vi "PrepareRollToPassReceiverGoToTactic.vi"(7 "first call":bool, 8 "error in (no error)":errorcluster, 9 "Game in":refnum<class "Game.lvclass">, 10 "Robot":refnum<class "Robot.lvclass">, 11 "PrepareRollToPassReceiverGoToTactic in":refnum<class "PrepareRollToPassReceiverGoToTactic.lvclass">) -> (0 "error out":errorcluster, 2 "Robot out":refnum<class "Robot.lvclass">, 3 "PrepareRollToPassReceiverGoToTactic out":refnum<class "PrepareRollToPassReceiverGoToTactic.lvclass">)   [LabVIEW 2023, in "PrepareRollToPassReceiverGoToTactic.lvclass"]
uses:
  PrepareRollToPassReceiverGoToTactic.lvclass
  Robot_class/Robot.lvclass
  Game_class/Game.lvclass
  Robot_class/tactics.ctl
  Tactic_class/Tactic.lvclass/Tactic.ctl
  Skillbook_class/Skillbook.lvclass/Skillbook.ctl
  Game_class/Game.lvclass/Game.ctl
  Object_class/Object.lvclass/Object.ctl
  Robot_class/Robot.lvclass/Robot.ctl
  PrepareRollToPassReceiverGoToTactic.lvclass/PrepareRollToPassReceiverGoToTactic.ctl
  <vilib>/Analysis/_algsub.llb/Real Vector Norm.vi
  Game_class/Read BallRef.vi
  Game_class/Read FieldRef.vi
  Object_class/Read x.vi
  Object_class/Read y.vi
  Skillbook_class/Read GoToSkill.vi
  Robot_class/Read orientation.vi
  Robot_class/Read dest_x.vi
  Robot_class/Read dest_y.vi
  Robot_class/Read dest_orientation.vi
  Tactic_class/Read Skillbook.vi
  Robot_class/Write tactic.vi
  Write States.vi
  Ball_class/Ball.lvclass
  Skillbook_class/Skillbook.lvclass
  Field_class/Field.lvclass
  GoToSkill_class/GoToSkill.lvclass
  <vilib>/Analysis/NI_AALPro.lvlib
panel:
  out "x .or. y?":bool
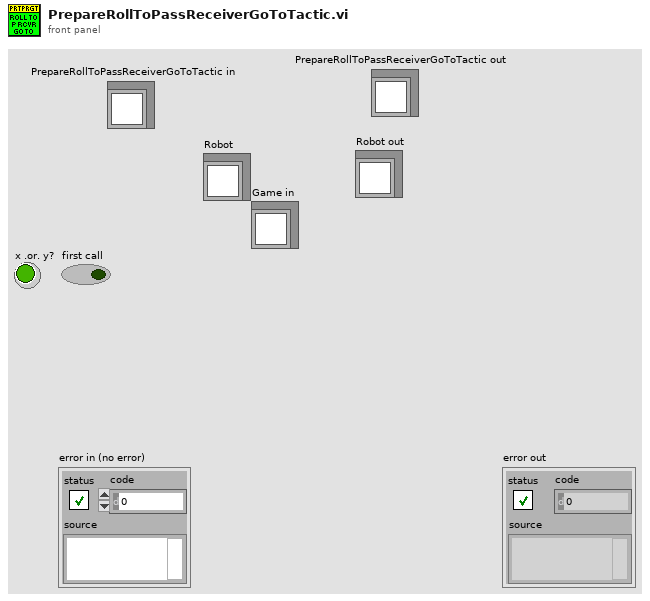
[diagram p1: front panel]
types:
  T1 = typedef "tactics.ctl" = enum16{"ReceivePassInFuturePoint", "Roller", "PrepareRollToPassRollerGoTo", "PrepareRollToPassReceiverGoTo", "WaitRoll", "PositionToRoll", "PenaltyAttacker", "PassObserver", "PenaltyDefense", "TableReceiverTactic", "Test", "DefendGoal", "Marker", "FollowAttacker", "DefendArea", "Shoot", "AttackerAimGoal", "AttackerBallOutOfField", "AttackerBlock", "AttackerStop", "Duelist", "Halt", "ZigZag", "GoTo", "Timeout", "KickToPassReceiver", "PositionToReceivePass", "DefendAreaVSS", "DefendGoalVSS", "KickVSS", "AttackVSS", "DispBallVSS", "PenaltyAttackVSS", "WaitPass"}
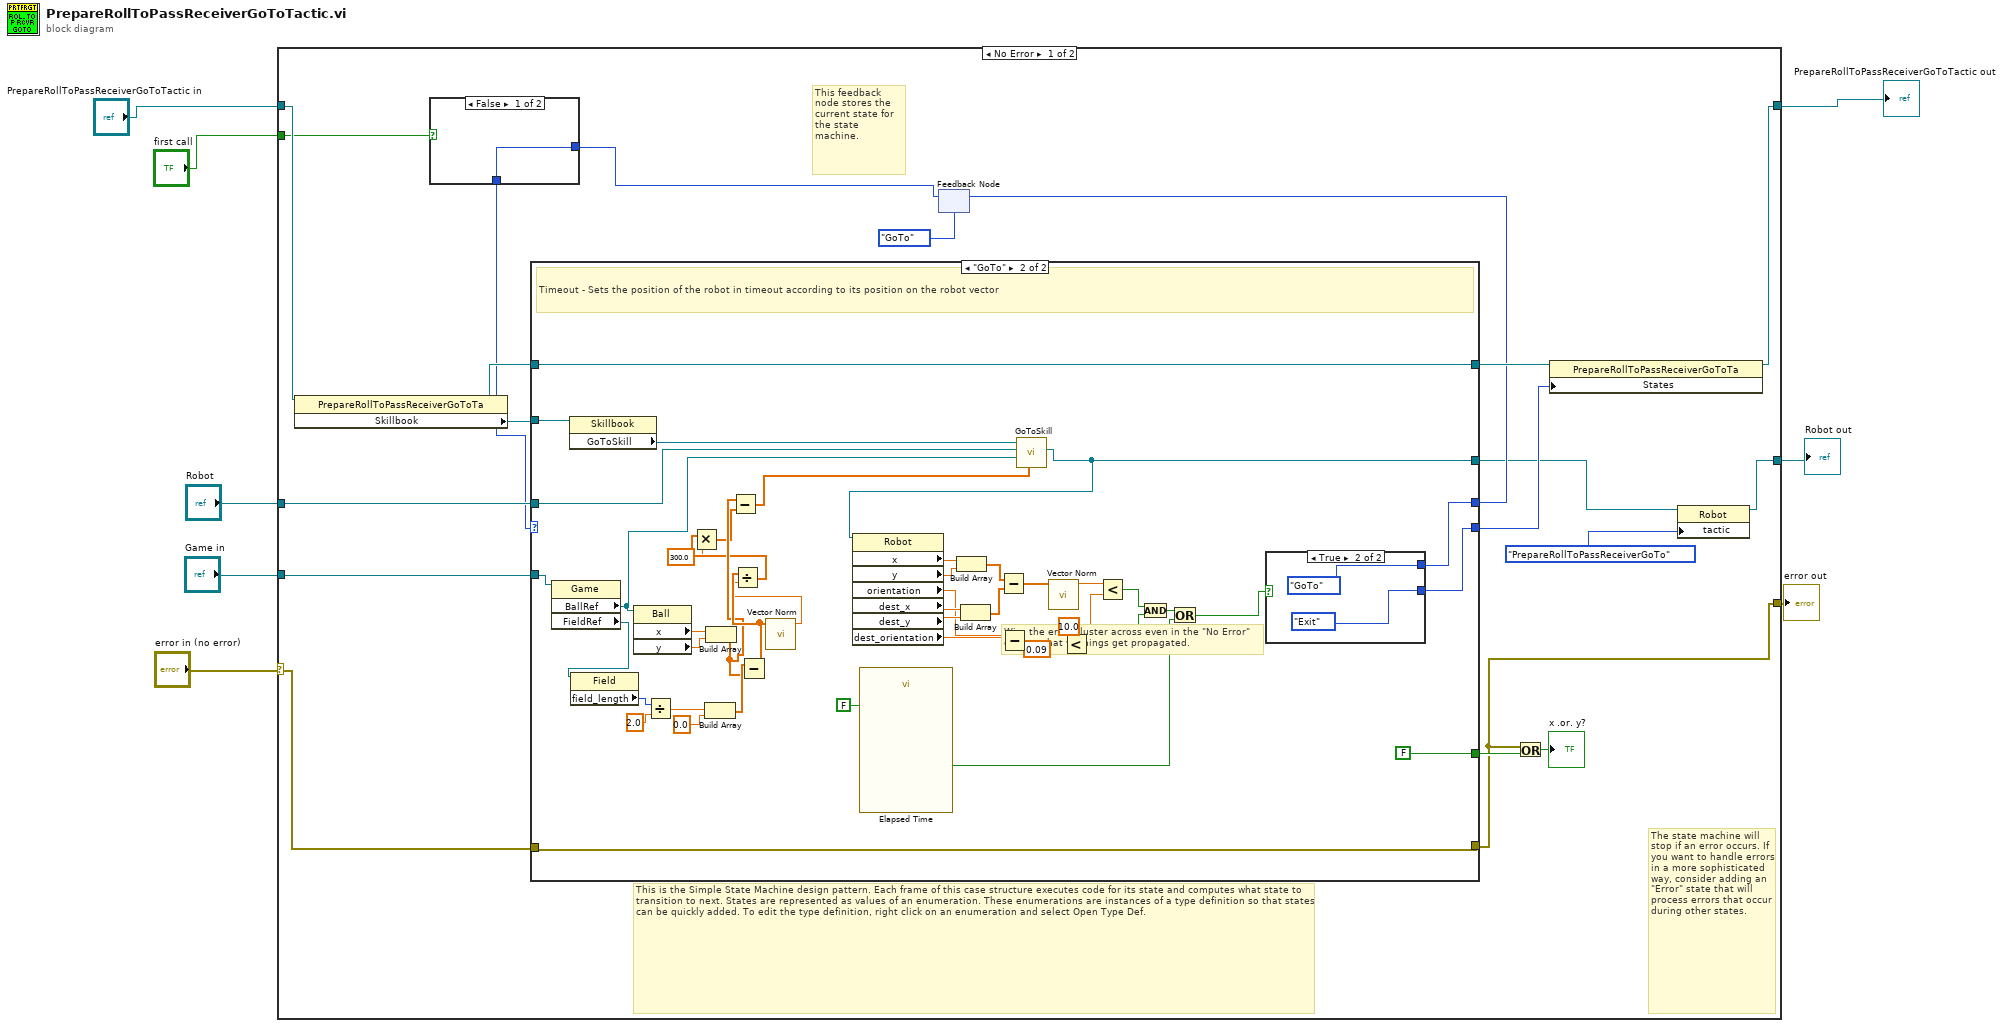
[diagram p0: block diagram]
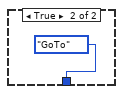
[diagram p2: hidden frame]
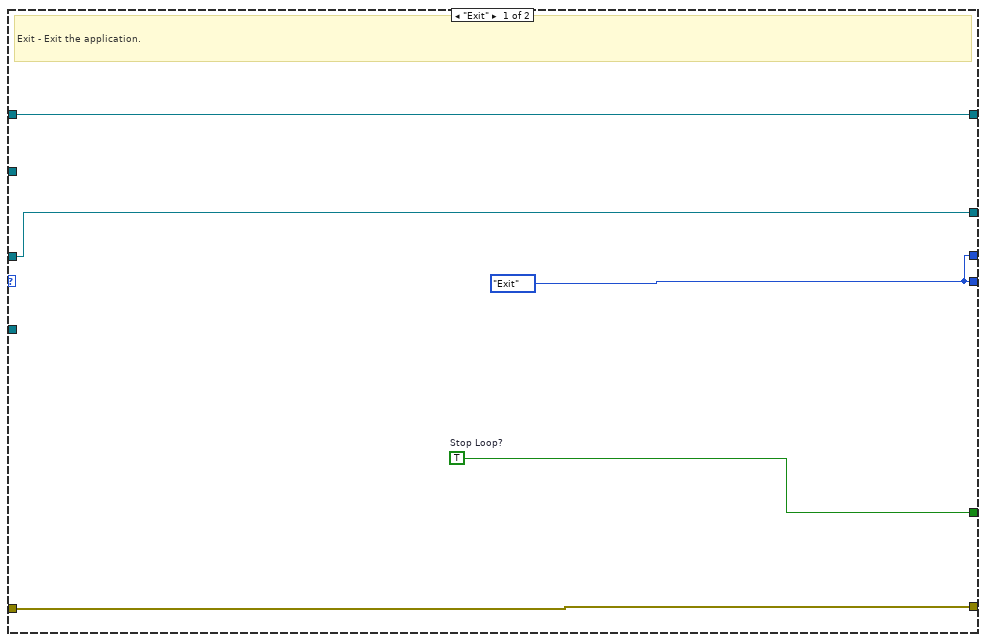
[diagram p3: hidden frame]
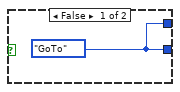
[diagram p4: hidden frame]
diagram:
  n1 = case shown="No Error" "error in (no error)" {
    selector: "error in (no error)" -> [w23 w86]
    tunnel: [w24 w86] -> w7
    tunnel: [w21 w85] -> w1
    tunnel: "PrepareRollToPassReceiverGoToTactic in" -> [w22 w85]
    tunnel: "Game in" -> [w19 _]
    tunnel: "Robot" -> [w18 w84]
    tunnel: [w10 w84] -> w5
    tunnel: "first call" -> [w15 _]
    frame No Error {
      # "The state machine will stop if an error occurs. If you want to handle errors in a more sophisticated way, consider adding an \"Error\" state that will process errors that occur during other states."
      # "This feedback node stores the current state for the state machine."
      # "This is the Simple State Machine design pattern. Each frame of this case structure executes code for its state and computes what state to transition to next. States are represented as values of an enumeration. These enumerations are instances of a type definition so that states can be quickly added. To edit the type definition, right click on an enumeration and select Open Type Def."
      # "Wire the error cluster across even in the \"No Error\"\ncase so that warnings get propagated."
      n2 = property class="PrepareRollToPassReceiverGoToTa"(reference=w22) -> (reference out=w20:refnum<class "PrepareRollToPassReceiverGoToTactic.lvclass">, "Skillbook"=w26:refnum<class "Skillbook.lvclass">)  [unwired: 1 in, 1 out]
      n3 = feedback #1(enum16{"Exit", "GoTo"}."GoTo" ("States")) -> (w13:enum16{"Exit", "GoTo"})
      n4 = case shown="False" w15 {
        tunnel: [w29 enum16{"Exit", "GoTo"}."GoTo" ("States")] -> w14
        tunnel: w13 -> [w29 _]
        frame False {
        }
        frame True {
        }
      }
      n5 = case shown="\"GoTo\"" w14 {
        tunnel: [w31 w76] -> w17
        tunnel: [w35 FALSE ("Stop Loop?")] -> w28
        tunnel: w23 -> [w34 w79]
        tunnel: [w34 w79] -> w24
        tunnel: w26 -> [_ w78]
        tunnel: w18 -> [w33 w53]
        tunnel: [w33 w54] -> w11
        tunnel: [w32 w77] -> w25
        tunnel: w20 -> [w32 w77]
        tunnel: w19 -> [_ w36]
        tunnel: [w31 w75] -> w16
        frame "Exit" {
          w31 = enum16{"Exit", "GoTo"}."Exit" ("States")
          w35 = TRUE  # Stop Loop?
          # "Exit - Exit the application."
        }
        frame "GoTo" {
          # "Timeout - Sets the position of the robot in timeout according to its position on the robot vector"
          n6 = property class="Game"(reference=w36) -> ("BallRef"=w37:refnum<class "Ball.lvclass">, "FieldRef"=w50:refnum<class "Field.lvclass">)  [unwired: 1 in, 2 out]
          n7 = property class="Skillbook"(reference=w78) -> ("GoToSkill"=w74:refnum<class "GoToSkill.lvclass">)  [unwired: 1 in, 2 out]
          n8 = property class="Field"(reference=w50) -> ("field_length"=w49:i32)  [unwired: 1 in, 2 out]
          n9 = property class="Ball"(reference=w37) -> ("x"=w52:dbl, "y"=w51:dbl)  [unwired: 1 in, 2 out]
          n10 = Divide(x=w49, y=2.0) -> (x/y=w47:dbl)
          n11 = Build Array(w47, 0.0) -> (w45:dbl[])
          n12 = Build Array(w52, w51) -> (w42:dbl[])
          n13 = Subtract(x=w45, y=w42) -> (x-y=w44:dbl[])
          n14 = call-poly <vilib>:"Vector Norm.vi"("Input Vector"=w44) -> ("norm"=w43:dbl)  [unwired: 9 in, 1 out]
          n15 = Divide(x=w44, y=w43) -> (x/y=w40:dbl[])
          n16 = Multiply(x=w40, y=300.0) -> (x*y=w41:dbl[])
          n17 = Subtract(x=w42, y=w41) -> (x-y=w38:dbl[])
          n18 = call "Elapsed Time"("Auto Reset"=FALSE) -> ("Time has Elapsed"=w56:bool)  [unwired: 11 in, 7 out]
          n19 = call "GoToSkill.vi"("Position"=w38, "BallRef"=w37, "Robot in"=w53, "GoToSkill in"=w74) -> ("Robot out"=w54:refnum<class "Robot.lvclass">)  [unwired: 5 in, 2 out]
          n20 = property class="Robot"(reference=w54) -> ("x"=w73:dbl, "y"=w72:dbl, "orientation"=w68:dbl, "dest_x"=w71:dbl, "dest_y"=w70:dbl, "dest_orientation"=w67:dbl)  [unwired: 1 in, 2 out]
          n21 = Build Array(w73, w72) -> (w55:dbl[])
          n22 = Build Array(w71, w70) -> (w69:dbl[])
          n23 = Subtract(x=w55, y=w69) -> (x-y=w66:dbl[])
          n24 = Subtract(x=w68, y=w67) -> (x-y=w63:dbl)
          n25 = call-poly <vilib>:"Vector Norm.vi"("Input Vector"=w66) -> ("norm"=w65:dbl)  [unwired: 9 in, 1 out]
          n26 = Less?(x=w63, y=0.09) -> (x < y?=w60:bool)
          n27 = Less?(x=w65, y=10.0) -> (x < y?=w61:bool)
          n28 = And(x=w61, y=w60) -> (x .and. y?=w58:bool)
          n29 = Or(x=w58, y=w56) -> (x .or. y?=w57:bool)
          n30 = case shown="True" w57 {
            tunnel: [w81 enum16{"Exit", "GoTo"}."Exit" ("States")] -> w76
            tunnel: [w81 enum16{"Exit", "GoTo"}."GoTo" ("States")] -> w75
            frame False {
              w81 = enum16{"Exit", "GoTo"}."GoTo" ("States")
            }
            frame True {
            }
          }
        }
      }
      n31 = feedback-in #1(w16) -> ()
      n32 = Or(x=w24, y=w28) -> (x .or. y?=→"x .or. y?":bool)
      n33 = property class="PrepareRollToPassReceiverGoToTa"(reference=w25, "States"=w17) -> (reference out=w21:refnum<class "PrepareRollToPassReceiverGoToTactic.lvclass">)  [unwired: 1 in, 1 out]
      n34 = property class="Robot"(reference=w11, "tactic"=tactics."PrepareRollToPassReceiverGoTo") -> (reference out=w10:refnum<class "Robot.lvclass">)  [unwired: 1 in, 1 out]
    }
    frame Error {
    }
  }
  "error out" <- w7
  "Robot out" <- w5
  "PrepareRollToPassReceiverGoToTactic out" <- w1
